vi "frequency demodulation.vi"(0 "signal":waveform(dbl), 1 "210Hz sine":waveform(dbl), 2 "210Hz cosine":waveform(dbl), 3 "500Hz sine":waveform(dbl), 4 "analog trigger in":waveform(dbl), 5 "500 Hz cosine":waveform(dbl)) -> (6 "blue":waveform(dbl), 7 "raw signal out":waveform(dbl), 8 "analog trig out":waveform(dbl), 9 "uv":waveform(dbl))   [LabVIEW 2013]
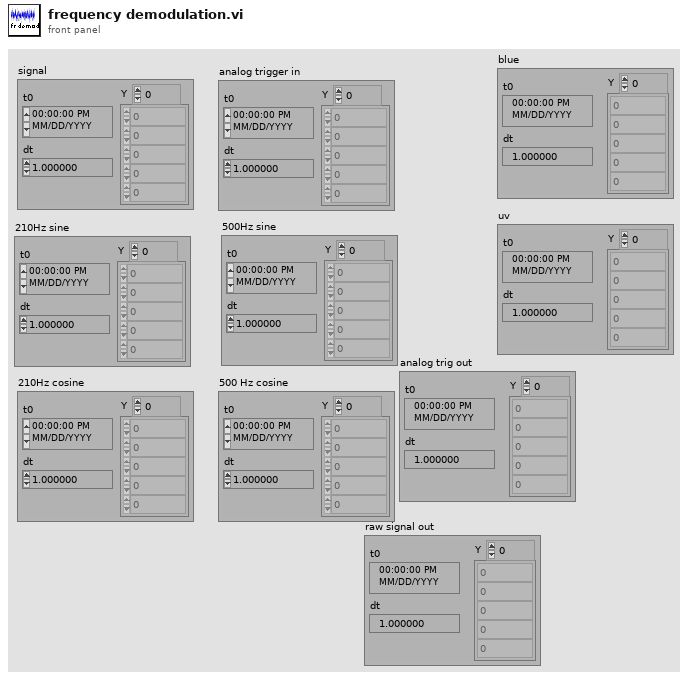
[diagram p1: front panel]
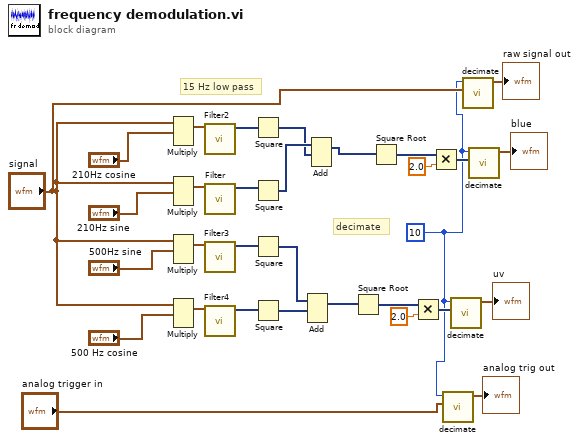
[diagram p0: block diagram]
diagram:
  w2 = 10 ("Divide by")
  # "15 Hz low pass"
  # "decimate"
  n1 = Multiply(1:"210Hz cosine", 2:"signal") -> (0:w30:waveform(dbl))  [unwired: 1 in, 1 out]
  n2 = Multiply(1:"210Hz sine", 2:"signal") -> (0:w31:waveform(dbl))  [unwired: 1 in, 1 out]
  n3 = Multiply(1:"500Hz sine", 2:"signal") -> (0:w21:waveform(dbl))  [unwired: 1 in, 1 out]
  n4 = Multiply(1:"500 Hz cosine", 2:"signal") -> (0:w20:waveform(dbl))  [unwired: 1 in, 1 out]
  n5 = call "Filter2"("Signal"=w30) -> ("Filtered Signal"=w28:dynamicdata)  [unwired: 9 in, 1 out]
  n6 = call "Filter"("Signal"=w31) -> ("Filtered Signal"=w29:dynamicdata)  [unwired: 9 in, 1 out]
  n7 = call "Filter3"("Signal"=w21) -> ("Filtered Signal"=w19:dynamicdata)  [unwired: 9 in, 1 out]
  n8 = call "Filter4"("Signal"=w20) -> ("Filtered Signal"=w18:dynamicdata)  [unwired: 9 in, 1 out]
  n9 = Square(x=w28) -> (x^2=w26:dynamicdata)
  n10 = Square(x=w29) -> (x^2=w27:dynamicdata)
  n11 = Square(x=w19) -> (x^2=w17:dynamicdata)
  n12 = Square(x=w18) -> (x^2=w16:dynamicdata)
  n13 = Add(1:w16, 2:w17) -> (0:w15:dynamicdata)  [unwired: 1 in, 1 out]
  n14 = Add(1:w26, 2:w27) -> (0:w25:dynamicdata)  [unwired: 1 in, 1 out]
  n15 = Square Root(x=w15) -> (sqrt(x)=w14:dynamicdata)
  n16 = Square Root(x=w25) -> (sqrt(x)=w24:dynamicdata)
  n17 = Multiply(x=w14, y=2.0) -> (x*y=w12:dynamicdata)
  n18 = Multiply(x=w24, y=2.0) -> (x*y=w22:dynamicdata)
  n19 = call "decimate.vi"("Waveform"="analog trigger in", "Divide by"=w2) -> ("output waveform"=→"analog trig out":waveform(dbl))  [unwired: 9 in]
  n20 = call "decimate.vi"("Waveform"=w12, "Divide by"=w2) -> ("output waveform"=→"uv":waveform(dbl))  [unwired: 9 in]
  n21 = call "decimate.vi"("Waveform"="signal", "Divide by"=w2) -> ("output waveform"=→"raw signal out":waveform(dbl))  [unwired: 9 in]
  n22 = call "decimate.vi"("Waveform"=w22, "Divide by"=w2) -> ("output waveform"=→"blue":waveform(dbl))  [unwired: 9 in]
